vi "Get Room State.vi"(8 "error in":errorcluster, 11 "Room In":refnum<class "Room.lvclass">) -> (0 "error out":errorcluster, 2 "Selected Room":T1={"RoomNumFlags"={"Room Number"=0, "Flag State"=[1, 3, 5, 7]}, "BedVacant"=FALSE, "InRoomPersonnel"=[], "RoomRequests"=[]}, 3 "Room Out":refnum<class "Room.lvclass">)   [LabVIEW 2015]
uses:
  Classes/Room/Room.lvclass
  TypeDef/SelectedRoom.ctl
  Classes/Room/Room.lvclass/Room.ctl
  Classes/Flags/Flags.lvclass
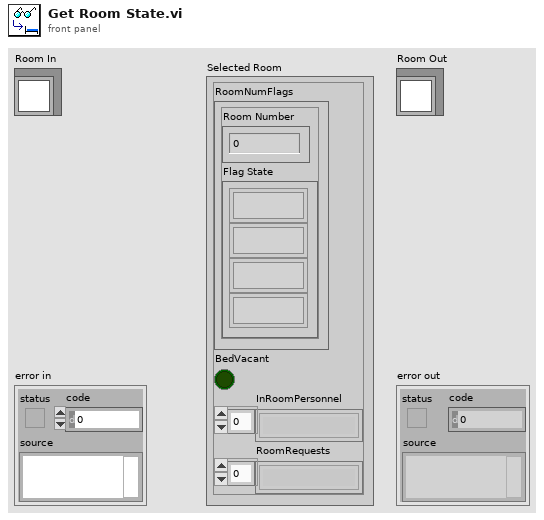
[diagram p1: front panel]
types:
  T1 = typedef "SelectedRoom.ctl" = cluster{"RoomNumFlags":cluster{"Room Number":u8, "Flag State":u8[]}, "BedVacant":bool, "InRoomPersonnel":string[], "RoomRequests":string[]}
  T2 = typedef "ColorFlags.ctl" = cluster{"Room Number":u32, "Flag State":u8[]}
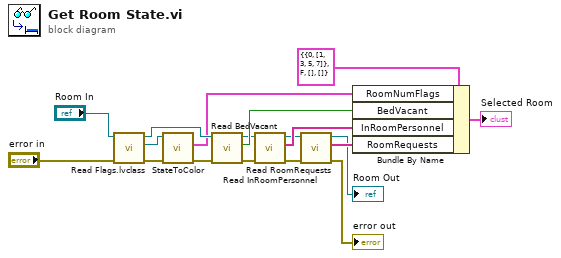
[diagram p0: block diagram]
diagram:
  n1 = call "Read Flags.lvclass.vi"("error in (no error)"="error in", "Room in"="Room In") -> ("error out"=w13:errorcluster, "Flags.lvclass"=w15:refnum<class "Flags.lvclass">, "Room out"=w16:refnum<class "Room.lvclass">)  [unwired: 7 in]
  n2 = call "StateToColor.vi"("error in (no error)"=w13, "Flags in"=w15) -> ("error out"=w12:errorcluster, "RoomNumFlags"=w14:T2)  [unwired: 7 in, 1 out]
  n3 = call "Read BedVacant.vi"("error in (no error)"=w12, "Room in"=w16) -> ("error out"=w10:errorcluster, "BedVacant"=w17:bool, "Room out"=w11:refnum<class "Room.lvclass">)  [unwired: 7 in]
  n4 = call "Read InRoomPersonnel.vi"("error in (no error)"=w10, "Room in"=w11) -> ("error out"=w8:errorcluster, "InRoomPersonnel"=w9:string[], "Room out"=w7:refnum<class "Room.lvclass">)  [unwired: 7 in]
  n5 = call "Read RoomRequests.vi"("error in (no error)"=w8, "Room in"=w7) -> ("error out"=→"error out":errorcluster, "RoomRequests"=w6:string[], "Room out"=→"Room Out":refnum<class "Room.lvclass">)  [unwired: 7 in]
  n6 = Bundle By Name(cluster=T1 {"RoomNumFlags"={"Room Number"=0, "Flag State"=[1, 3, 5, 7]}, "BedVacant"=FALSE, "InRoomPersonnel"=[], "RoomRequests"=[]} ("Selected Room"), "RoomNumFlags"=w14, "BedVacant"=w17, "InRoomPersonnel"=w9, "RoomRequests"=w6) -> (→"Selected Room":T1)
